vi "复位定时器.vi"(8 "error in (no error)":errorcluster caption="错误输入（无错误）", 11 "定时器 输入":refnum<class "定时器.lvclass">) -> (0 "error out":errorcluster caption="错误输出", 3 "定时器 输出":refnum<class "定时器.lvclass">)   [LabVIEW 2017, in "定时器.lvclass"]
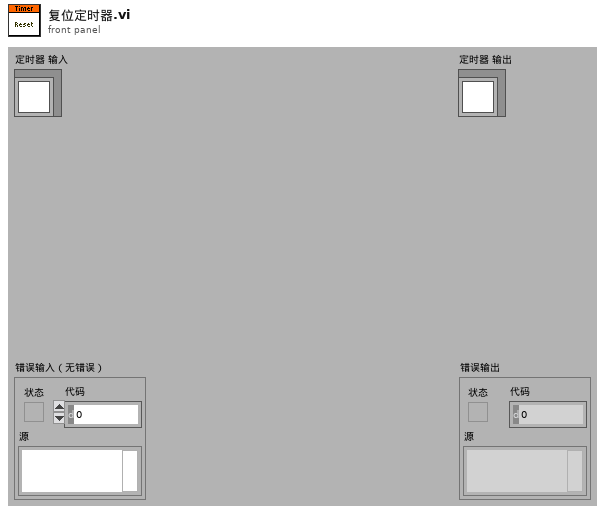
[diagram p1: front panel]
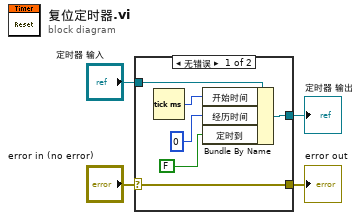
[diagram p0: block diagram]
diagram:
  n1 = case shown="无错误" "error in (no error)" {
    selector: "error in (no error)" -> [w10 w12]
    tunnel: [w10 w12] -> w3
    tunnel: [w7 w11] -> w1
    tunnel: "定时器 输入" -> [w9 w11]
    frame No Error {
      n2 = Tick Count (ms)() -> (millisecond timer value=w8:u32)
      n3 = Bundle By Name(cluster=w9, "开始时间"=w8, "经历时间"=u32 0, "定时到"=FALSE) -> (w7:refnum<class "定时器.lvclass">)
    }
    frame Error {
    }
  }
  "error out" <- w3
  "定时器 输出" <- w1
